vi "Read value 2.vi"(8 "error in (no error)":errorcluster, 11 "DataLogging in":refnum<class "DataLogging.lvclass">) -> (0 "error out":errorcluster, 2 "value 2":dbl, 3 "DataLogging out":refnum<class "DataLogging.lvclass">)   [LabVIEW 2017, in "DataLogging.lvclass"]
uses:
  DataLogging.lvclass
  DataLogging.lvclass/DataLogging.ctl
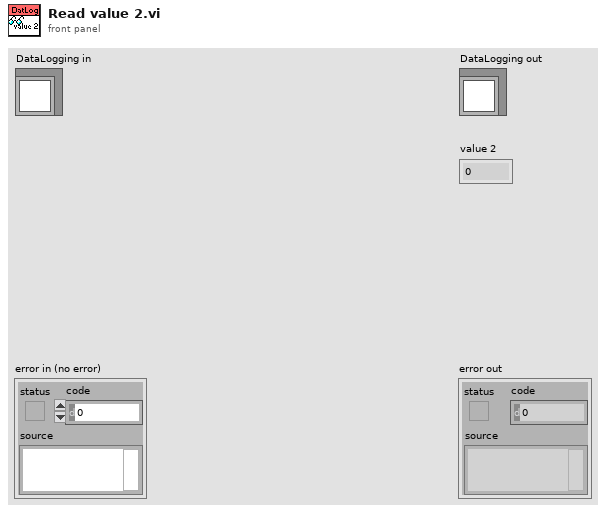
[diagram p1: front panel]
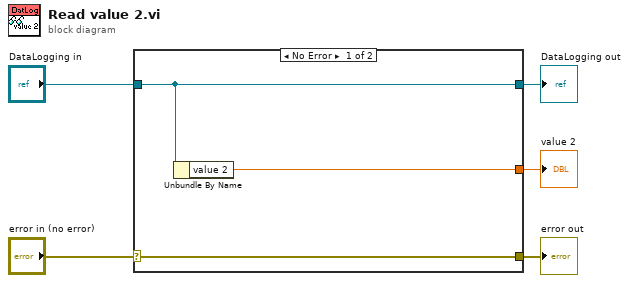
[diagram p0: block diagram]
diagram:
  n1 = case shown="No Error" "error in (no error)" {
    selector: "error in (no error)" -> [w8 w9]
    tunnel: [w8 w9] -> w4
    tunnel: [w7 w10] -> w2
    tunnel: "DataLogging in" -> [w7 w10]
    tunnel: [w6 _] -> w1
    frame No Error {
      n2 = Unbundle By Name(w7) -> ("value 2"=w6:dbl)
    }
    frame Error {
    }
  }
  "error out" <- w4
  "DataLogging out" <- w2
  "value 2" <- w1
